vi "next chunk - read-write freq PID file - atomic actions .vi"(0 "sweep folder path":path, 1 "PID action":T2, 2 "ctl kind IN":T1, 3 "ctl kind OUT":T1, 5 "PID freq IN":dbl[](array[numeric]), 7 "temperatures IN":dbl[](array[numeric]), 9 "frequencies IN":dbl[][](array[numeric]), 11 "header IN":string[](array[string]), 12 "temperature":dbl, 13 "weights":dbl[](array[numeric]), 14 "frequency":dbl) -> (4 "sweep folder path out":path, 6 "PID freq":dbl[](array[numeric]), 8 "temperatures":dbl[](array[numeric]), 10 "frequencies":dbl[][](array[numeric]), 15 "header":string[](array[string]))   [LabVIEW 2015]
uses:
  next chunk read-write PID -- action.ctl
  ctl -- name dispatcher -- action.ctl
  Q -- check range -- i -- real.vi
  Q - not nan -- real.vi
  <vilib>/gmath/function.llb/Binomial Coefficient.vi
  <vilib>/Utility/file.llb/Write To Spreadsheet File (string).vi
  <vilib>/Utility/libraryn.llb/Check if File or Folder Exists.vi
panel:
  in  "significant digits":i32=10000
  out "number":i32=9
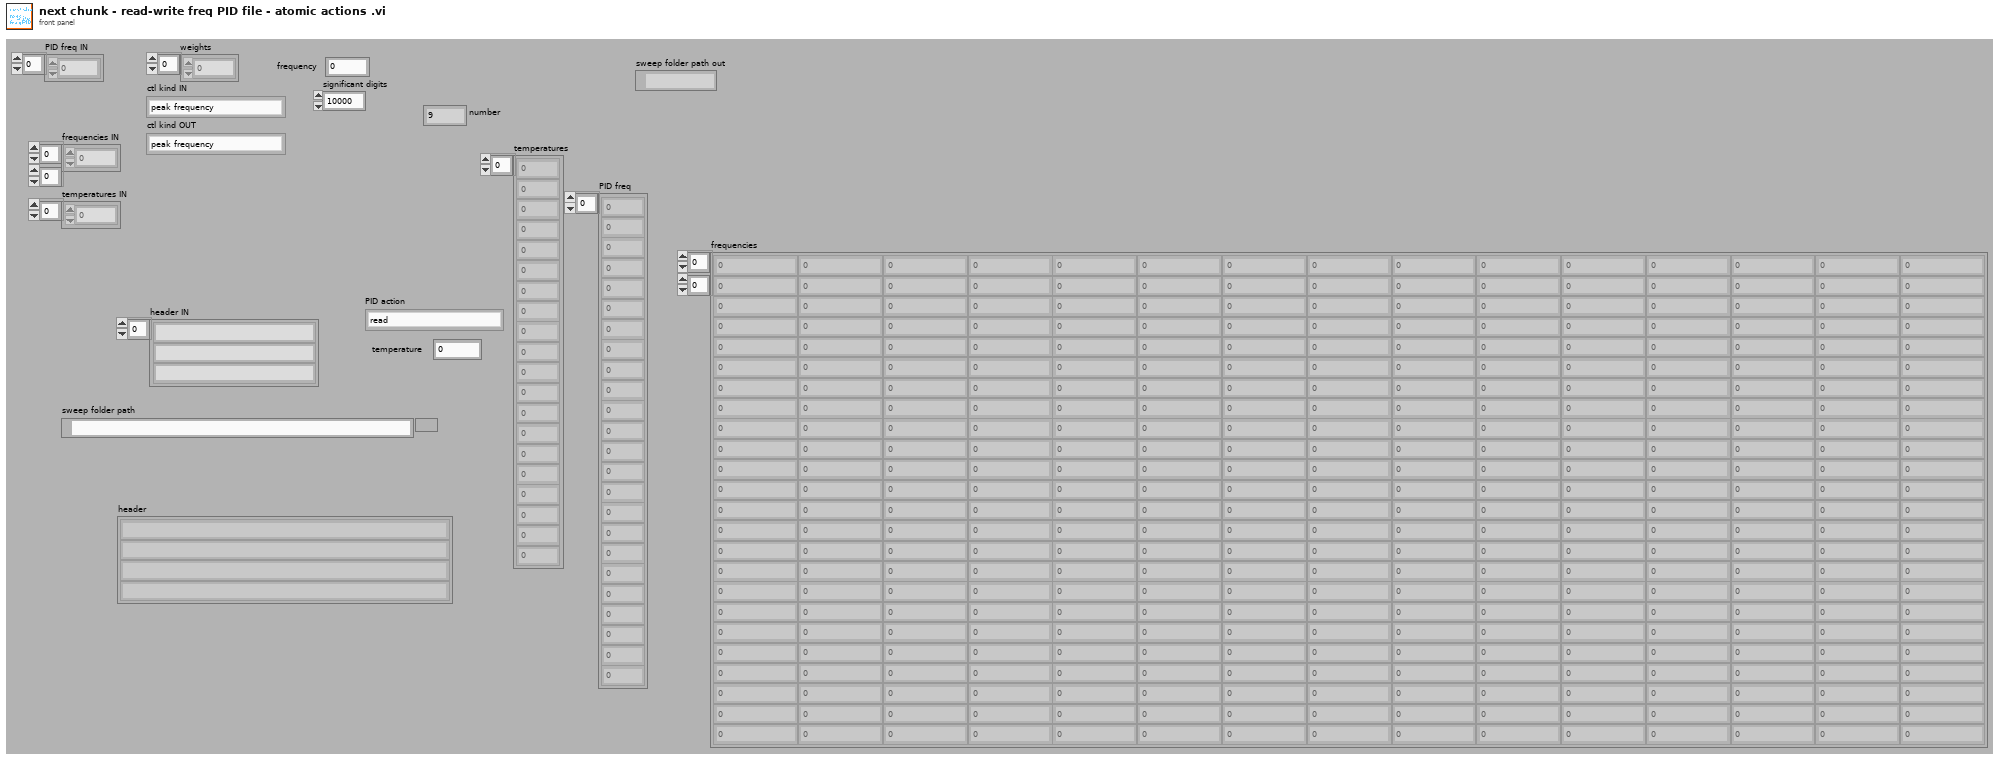
[diagram p1: front panel]
types:
  T1 = typedef "ctl -- name dispatcher -- action.ctl" = enum16{"peak frequency", "peak frequency DUMP", "peak gamma DUMP", "peak gamma", "peak frequency TEST", "peak gamma TEST", "ultrasonic power", "time in gamma", "set temperature ", "set temperature timer", "peak default gamma", "last scan file", "peak freq gamma TEST", "peak NAMES", "errors", "P_I_D", "P", "I", "D", "power vs time", "power vs time TIMER", "void", "power log", "set temperature - SINE", "itc ltc log", "peak - time in gamma"}
  T2 = typedef "next chunk read-write PID -- action.ctl" = enum16{"read", "interpolate", "append col", "write", "write PID col", "append PID col", "interpolate - bezier"}
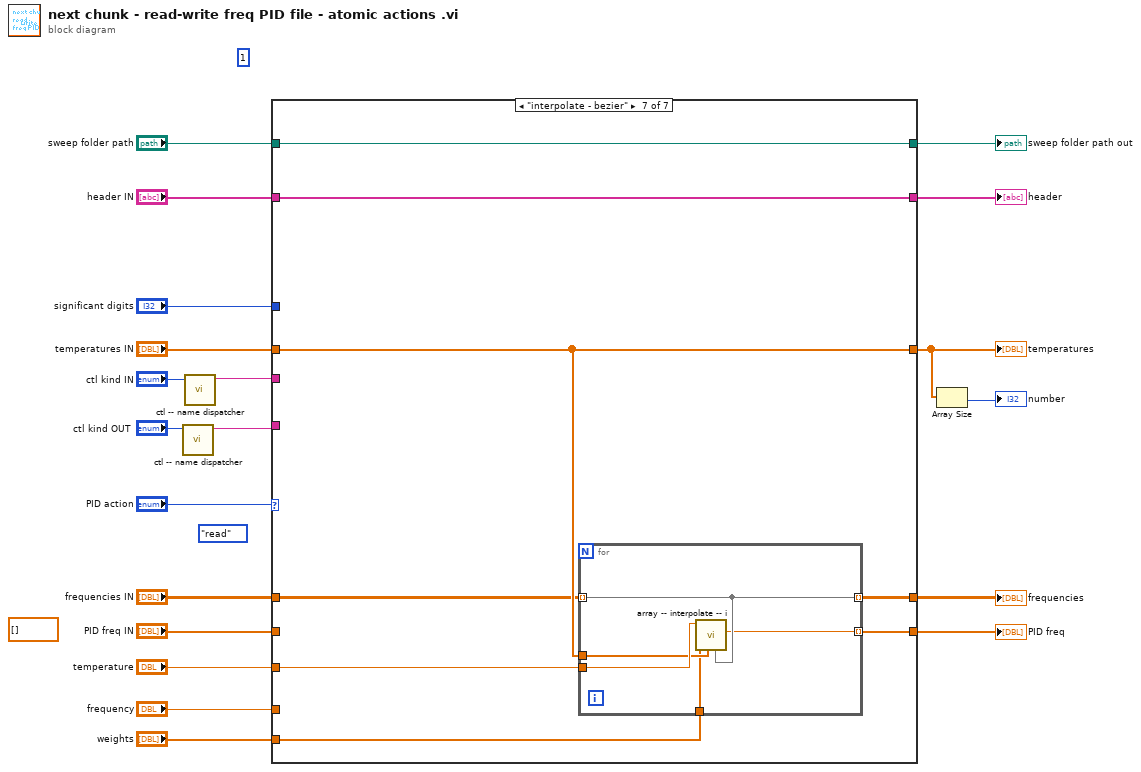
[diagram p0: block diagram]
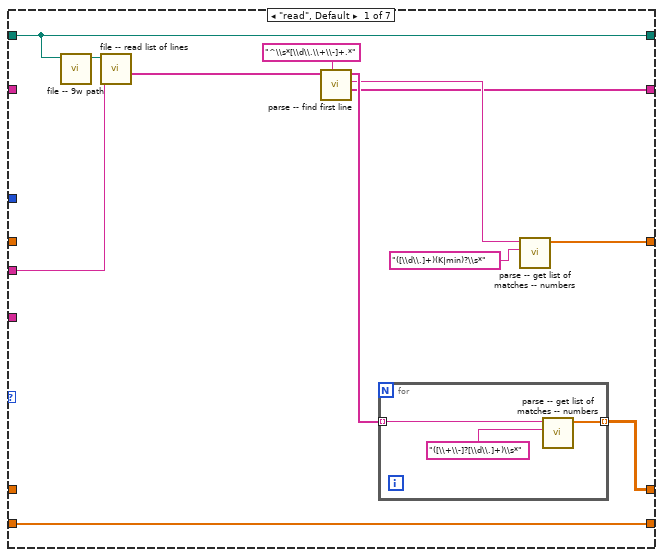
[diagram p2: hidden frame]
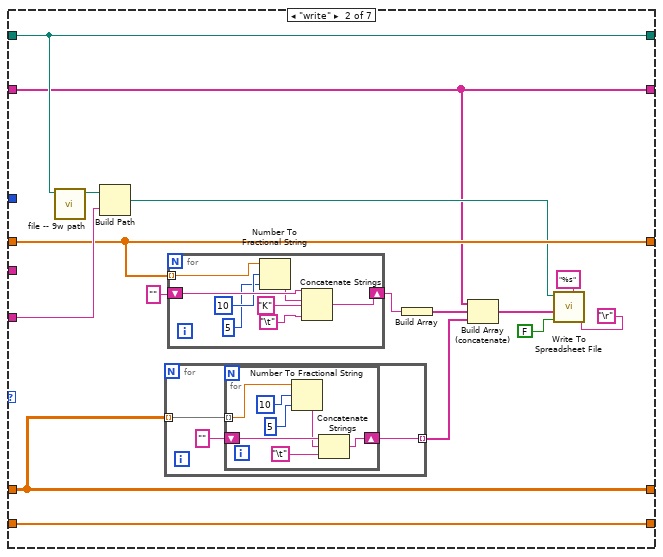
[diagram p3: hidden frame]
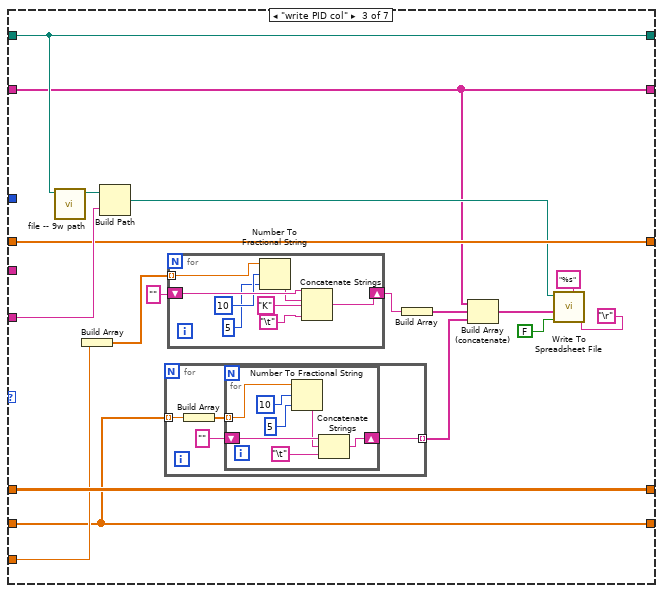
[diagram p4: hidden frame]
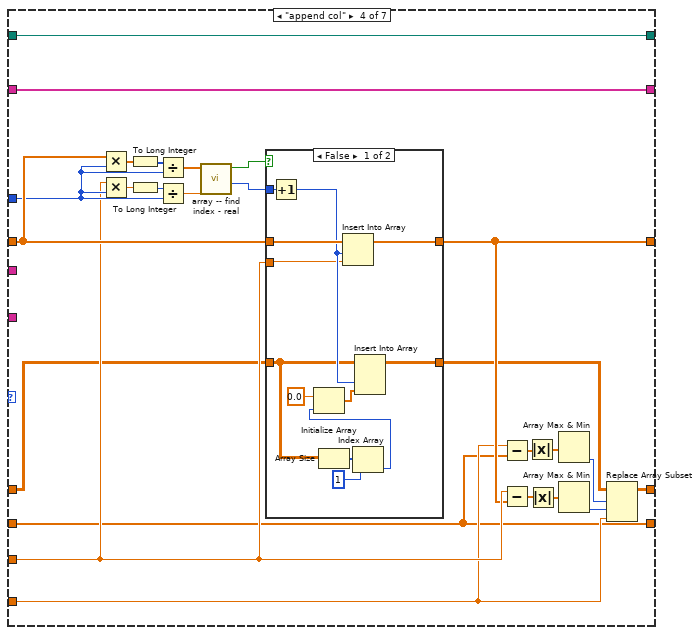
[diagram p5: hidden frame]
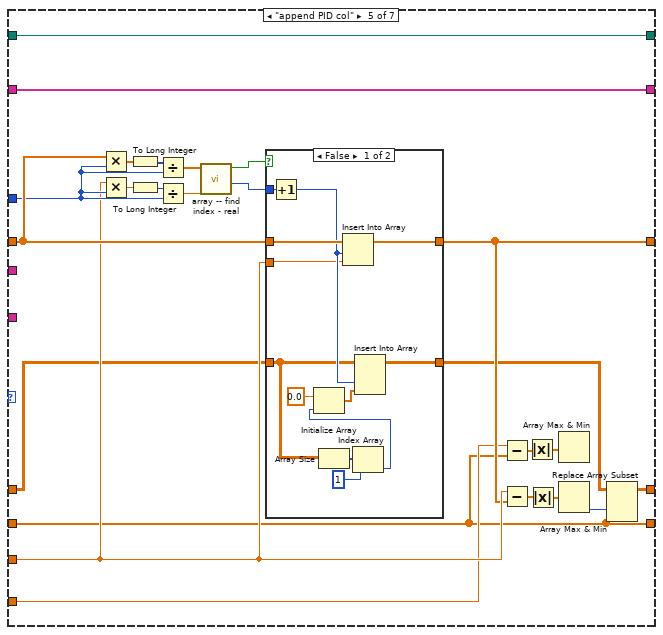
[diagram p7: hidden frame]
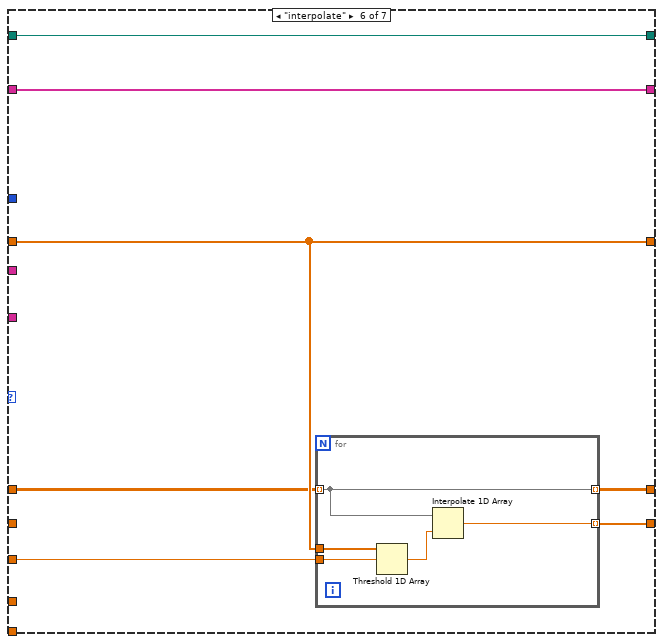
[diagram p9: hidden frame]
diagram:
  (unwired) dbl[] []
  (unwired) next_chunk_read-write_PID_--_action."read" ("PID action")
  (unwired) 1
  n1 = call "ctl -- name dispatcher.vi"("ctl name dispatch"="ctl kind OUT") -> ("ctl file name"=w1:string)  [unwired: 8 in, 2 out]
  n2 = call "ctl -- name dispatcher.vi"("ctl name dispatch"="ctl kind IN") -> ("ctl file name"=w3:string)  [unwired: 8 in, 2 out]
  n3 = case shown="\"interpolate - bezier\"" "PID action" {
    tunnel: [w32 w41 w78 w115 w154 w190 w203] -> w20
    tunnel: "temperature" -> [_ _ w72 w117 w156 w189 w202]
    tunnel: [w30 w50 w70 w107 w146 w188 w197] -> w18
    tunnel: "sweep folder path" -> [w29 w40 w77 w109 w148 w185 w199]
    tunnel: w3 -> [w22 _ _ _ _ _ _]
    tunnel: [w28 w47 w84 w114 w153 w187 w201] -> w15
    tunnel: "temperatures IN" -> [_ w47 w84 w120 w159 w187 w201]
    tunnel: "frequencies IN" -> [_ w41 w78 w116 w155 w186 w200]
    tunnel: "PID freq IN" -> [w30 w50 w70 w107 w146 _ _]
    tunnel: w1 -> [_ w49 w86 _ _ _ _]
    tunnel: "frequency" -> [_ _ _ w110 w149 _ _]
    tunnel: [w29 w40 w77 w109 w148 w185 w199] -> w12
    tunnel: [w24 w39 w76 w108 w147 w184 w198] -> w9
    tunnel: "header IN" -> [_ w39 w76 w108 w147 w184 w198]
    tunnel: "significant digits" -> [_ _ _ w119 w158 _ _]
    tunnel: "weights" -> [_ _ _ _ _ _ w196]
    frame "read", Default {
      n4 = call "file -- 9w path.vi"("sweep folder"=w29) -> ("9w path"=w23:path)  [unwired: 10 in]
      n5 = call "file -- read list of lines.vi"("file name"=w22, "folder path"=w23) -> ("text lines"=w21:string[])  [unwired: 9 in]
      n6 = call "parse -- find first line.vi"("regexp"="^\\s*[\\d\\.\\+\\-]+.*", "string array"=w21) -> ("before"=w24:string[], "matching line"=w25:string, "after"=w26:string[])  [unwired: 5 in, 2 out]
      n7 = for {
        tunnel: [w34] -> w32 mode=indexing
        tunnel: w26 -> [w33] mode=indexing
        n8 = call "parse -- get list of matches -- numbers.vi"("regexp"="([\\+\\-]?[\\d\\.]+)\\s*", "string"=w33) -> ("Array of numbers"=w34:dbl[])  [unwired: 6 in, 3 out]
      }
      n9 = call "parse -- get list of matches -- numbers.vi"("regexp"="([\\d\\.]+)(K|min)?\\s*", "string"=w25) -> ("Array of numbers"=w28:dbl[])  [unwired: 6 in, 3 out]
    }
    frame "write" {
      n10 = call "file -- 9w path.vi"("sweep folder"=w40) -> ("9w path"=w51:path)  [unwired: 10 in]
      n11 = Build Path(base path=w51, name or relative path=w49) -> (appended path=w42:path)
      n12 = for {
        tunnel: w41 -> [w61] mode=indexing
        tunnel: [w60] -> w37 mode=indexing
        n13 = for {
          tunnel: w61 -> [w69] mode=indexing
          shift-right: [w67] -> w60
          shift-left: "" ("format (%s)") -> [w68]
          n14 = Number To Fractional String(number=w69, width (-)=i16 10, precision (6)=i16 5 ("width (-)")) -> (F-format string=w66:string)  [unwired: 1 in]
          n15 = Concatenate Strings(w68, w66, "\t") -> (w67:string)
        }
      }
      n16 = for {
        tunnel: w47 -> [w55] mode=indexing
        shift-right: [w58] -> w43
        shift-left: "" ("format (%s)") -> [w59]
        n17 = Number To Fractional String(number=w55, width (-)=i16 10, precision (6)=i16 5 ("width (-)")) -> (F-format string=w52:string)  [unwired: 1 in]
        n18 = Concatenate Strings(w59, w52, "K" ("format (%s)"), "\t") -> (w58:string)
      }
      n19 = Build Array(w43) -> (w38:string[])
      n20 = Build Array (concatenate)(w39, w38, w37) -> (w36:string[])
      n21 = call-poly <vilib>:"Write To Spreadsheet File.vi"("delimiter (\\t)"="\r", "format (%s)"="%s", "append to file? (new file:F)"=FALSE, "1D data"=w36, "file path (dialog if empty)"=w42) -> ()  [unwired: 3 in, 1 out]
    }
    frame "write PID col" {
      n22 = call "file -- 9w path.vi"("sweep folder"=w77) -> ("9w path"=w87:path)  [unwired: 10 in]
      n23 = Build Array(w72) -> (w71:dbl[])
      n24 = Build Path(base path=w87, name or relative path=w86) -> (appended path=w79:path)
      n25 = for {
        tunnel: w70 -> [w97] mode=indexing
        tunnel: [w98] -> w74 mode=indexing
        n26 = Build Array(w97) -> (w96:dbl[])
        n27 = for {
          tunnel: w96 -> [w106] mode=indexing
          shift-right: [w104] -> w98
          shift-left: "" ("format (%s)") -> [w105]
          n28 = Number To Fractional String(number=w106, width (-)=i16 10, precision (6)=i16 5 ("width (-)")) -> (F-format string=w103:string)  [unwired: 1 in]
          n29 = Concatenate Strings(w105, w103, "\t") -> (w104:string)
        }
      }
      n30 = for {
        tunnel: w71 -> [w91] mode=indexing
        shift-right: [w94] -> w80
        shift-left: "" ("format (%s)") -> [w95]
        n31 = Number To Fractional String(number=w91, width (-)=i16 10, precision (6)=i16 5 ("width (-)")) -> (F-format string=w88:string)  [unwired: 1 in]
        n32 = Concatenate Strings(w95, w88, "K" ("format (%s)"), "\t") -> (w94:string)
      }
      n33 = Build Array(w80) -> (w75:string[])
      n34 = Build Array (concatenate)(w76, w75, w74) -> (w73:string[])
      n35 = call-poly <vilib>:"Write To Spreadsheet File.vi"("delimiter (\\t)"="\r", "format (%s)"="%s", "append to file? (new file:F)"=FALSE, "1D data"=w73, "file path (dialog if empty)"=w79) -> ()  [unwired: 3 in, 1 out]
    }
    frame "append col" {
      n36 = Multiply(x=w120, y=w119) -> (x*y=w122:dbl[])
      n37 = Multiply(x=w117, y=w119) -> (x*y=w125:dbl)
      n38 = To Long Integer(number=w122) -> (32bit integer=w121:i32[])
      n39 = To Long Integer(number=w125) -> (32bit integer=w124:i32)
      n40 = Divide(x=w121, y=w119) -> (x/y=w118:dbl[])
      n41 = Divide(x=w124, y=w119) -> (x/y=w123:dbl)
      n42 = call "array -- find index - real.vi"("number"=w123, "temperatures"=w118) -> ("left index"=w131:i32, "exact match ?"=w126:bool)  [unwired: 6 in, 2 out]
      n43 = case shown="False" w126 {
        tunnel: [w134 w144] -> w113
        tunnel: [w142 w145] -> w114
        tunnel: w120 -> [w143 w145]
        tunnel: w117 -> [w137 _]
        tunnel: w131 -> [w136 _]
        tunnel: w116 -> [w135 w144]
        frame False {
          n44 = Increment(x=w136) -> (x+1=w138:i32)
          n45 = Array Size(array=w135) -> (size(s)=w133:i32[])
          n46 = Insert Into Array(array=w143, index=w138, new element=w137) -> (w142:dbl[])
          n47 = Index Array(array=w133, index=1) -> (element=w132:i32)
          n48 = Initialize Array(0.0 ("element"), w132) -> (w141:dbl[])
          n49 = Insert Into Array(array=w135, index (col)=w138, new element=w141) -> (w134:dbl[][])  [unwired: 1 in]
        }
        frame True {
        }
      }
      n50 = Subtract(x=w110, y=w107) -> (x-y=w127:dbl[])
      n51 = Subtract(x=w117, y=w114) -> (x-y=w129:dbl[])
      n52 = Absolute Value(x=w127) -> (abs(x)=w111:dbl[])
      n53 = Absolute Value(x=w129) -> (abs(x)=w128:dbl[])
      n54 = Array Max & Min(array=w111) -> (min index (indices)=w130:i32)  [unwired: 3 out]
      n55 = Array Max & Min(array=w128) -> (min index (indices)=w112:i32)  [unwired: 3 out]
      n56 = Replace Array Subset(array=w113, new element=w110, index (row)=w130, index (col)=w112) -> (w115:dbl[][])
    }
    frame "append PID col" {
      n57 = Multiply(x=w159, y=w158) -> (x*y=w161:dbl[])
      n58 = Multiply(x=w156, y=w158) -> (x*y=w164:dbl)
      n59 = To Long Integer(number=w161) -> (32bit integer=w160:i32[])
      n60 = To Long Integer(number=w164) -> (32bit integer=w163:i32)
      n61 = Divide(x=w160, y=w158) -> (x/y=w157:dbl[])
      n62 = Divide(x=w163, y=w158) -> (x/y=w162:dbl)
      n63 = call "array -- find index - real.vi"("number"=w162, "temperatures"=w157) -> ("left index"=w169:i32, "exact match ?"=w165:bool)  [unwired: 6 in, 2 out]
      n64 = case shown="False" w165 {
        tunnel: [w172 w182] -> w152
        tunnel: [w180 w183] -> w153
        tunnel: w159 -> [w181 w183]
        tunnel: w156 -> [w175 _]
        tunnel: w169 -> [w174 _]
        tunnel: w155 -> [w173 w182]
        frame False {
          n65 = Increment(x=w174) -> (x+1=w176:i32)
          n66 = Array Size(array=w173) -> (size(s)=w171:i32[])
          n67 = Insert Into Array(array=w181, index=w176, new element=w175) -> (w180:dbl[])
          n68 = Index Array(array=w171, index=1) -> (element=w170:i32)
          n69 = Initialize Array(0.0 ("element"), w170) -> (w179:dbl[])
          n70 = Insert Into Array(array=w173, index (col)=w176, new element=w179) -> (w172:dbl[][])  [unwired: 1 in]
        }
        frame True {
        }
      }
      n71 = Subtract(x=w149, y=w146) -> (x-y=w166:dbl[])
      n72 = Subtract(x=w156, y=w153) -> (x-y=w168:dbl[])
      n73 = Absolute Value(x=w166) -> (abs(x)=w150:dbl[])
      n74 = Absolute Value(x=w168) -> (abs(x)=w167:dbl[])
      n75 = Array Max & Min(array=w150) -> ()  [unwired: 4 out]
      n76 = Array Max & Min(array=w167) -> (min index (indices)=w151:i32)  [unwired: 3 out]
      n77 = Replace Array Subset(array=w152, new element=w146, index (col)=w151) -> (w154:dbl[][])  [unwired: 1 in]
    }
    frame "interpolate" {
      n78 = for {
        tunnel: [w193] -> w190 mode=indexing
        tunnel: w187 -> [w191]
        tunnel: w189 -> [w192]
        tunnel: [w194] -> w188 mode=indexing
        tunnel: w186 -> [w193] mode=indexing
        n79 = Threshold 1D Array(2:w192, 3:w191) -> (0:w195:dbl)  [unwired: 1 in]
        n80 = Interpolate 1D Array(1:w195, 2:w193) -> (0:w194:dbl)
      }
    }
    frame "interpolate - bezier" {
      n81 = for {
        tunnel: [w206] -> w203 mode=indexing
        tunnel: w201 -> [w207]
        tunnel: w202 -> [w208]
        tunnel: w200 -> [w206] mode=indexing
        tunnel: [w205] -> w197 mode=indexing
        tunnel: w196 -> [w204]
        n82 = call "array -- interpolate -- i.vi"("all Voltage"=w206, "all tempearure"=w207, "weights"=w204, "temperature (K)"=w208) -> ("V out"=w205:dbl)  [unwired: 7 in]
      }
    }
  }
  "frequencies" <- w20
  "temperatures" <- w15
  "PID freq" <- w18
  "sweep folder path out" <- w12
  "header" <- w9
  n83 = Array Size(array=w15) -> (size(s)=→"number":i32)
